vi "e.gate HighSpeedPort Get File - Read Directory.vi"(7 "Timeout (ms) [1000]":i32=1000, 8 "error in (no error)":errorcluster, 10 "Drive Index":T1(ring), 11 "Configuration in":T2) -> (0 "error out":errorcluster, 2 "data out":string[](array[string]), 3 "Configuration out":T2)   [LabVIEW 2016]
uses:
  e.gate Configuration.ctl
  e.gate Channel Data.ctl
  e.gate Data Type.ctl
  e.gate Protocol Type.ctl
  e.gate Module  Data.ctl
  e.gateHSP_DLLhandle.ctl
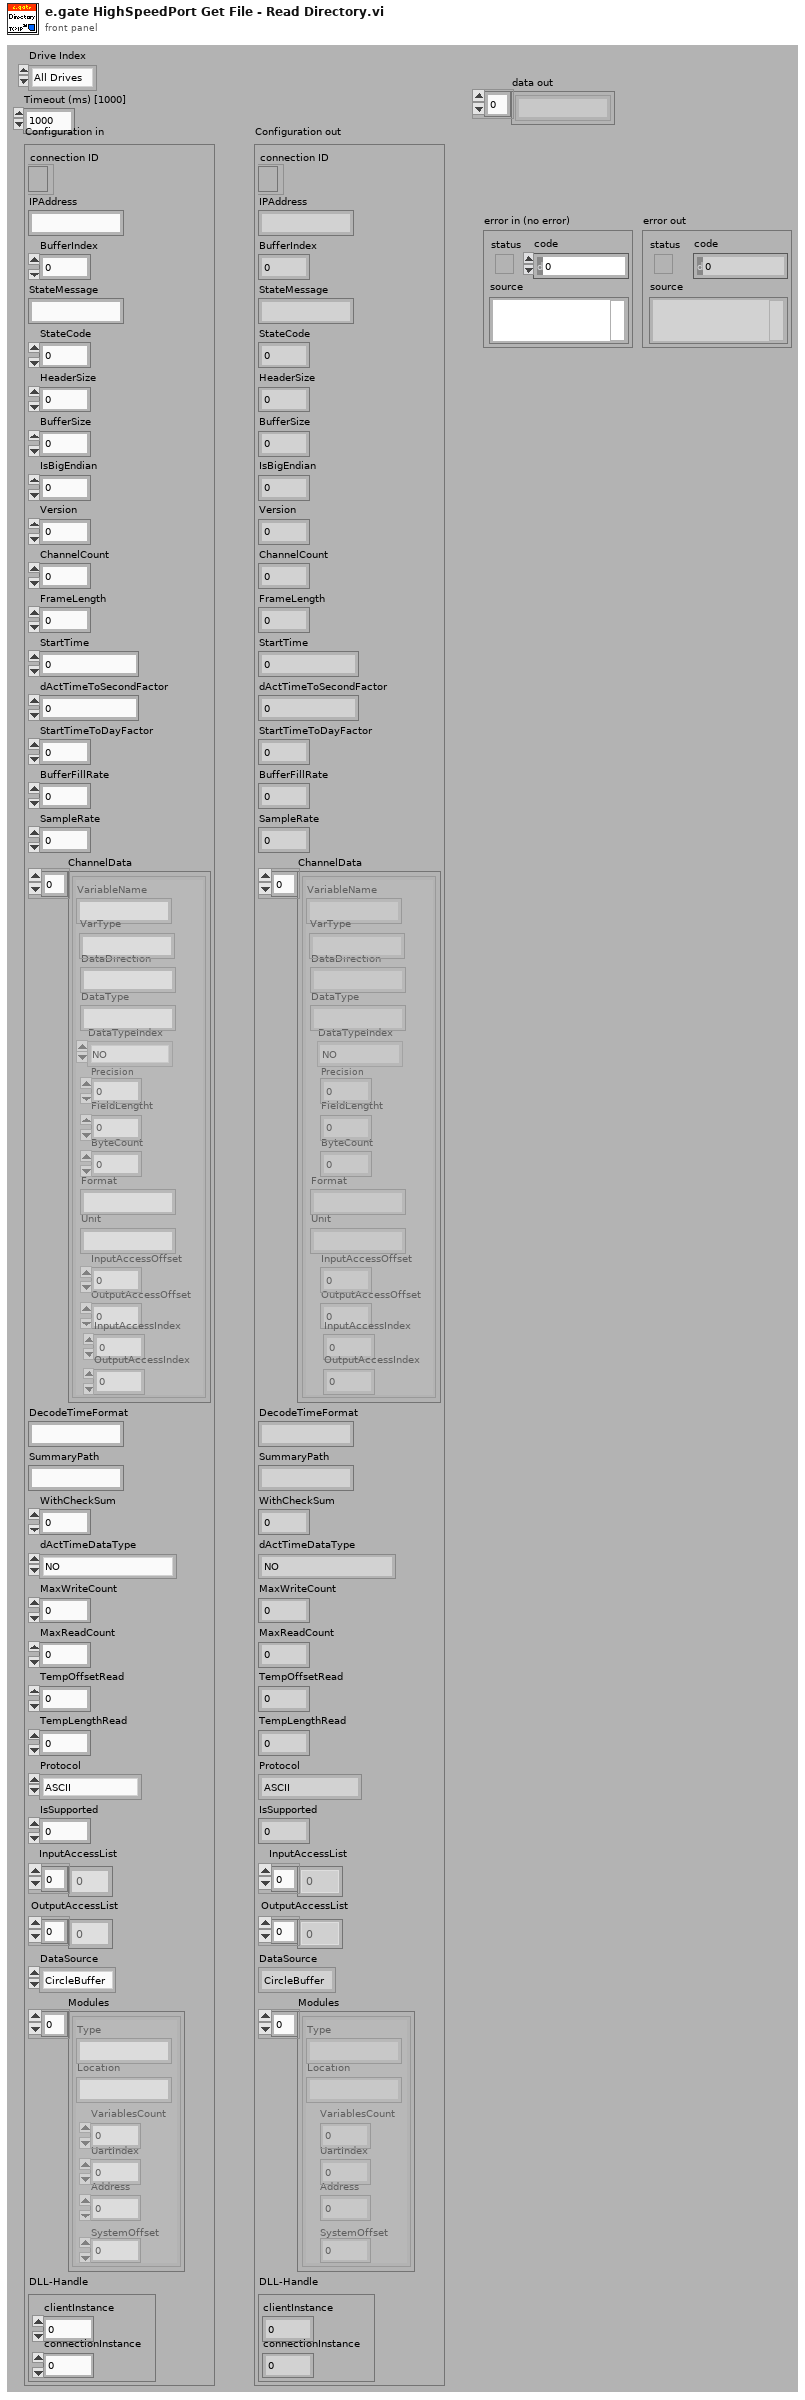
[diagram p1: front panel]
types:
  T1 = enum16{"All Drives", "Flash - Application Files", "Flash - Data", "USB Storage - Data", "Virtual State", "Virtual Circlebuffer", "Virtual Onlinebuffer", "Virtual Archive", "Virtual Logger"}
  T2 = typedef "e.gate Configuration.ctl" = cluster{"connection ID":refnum<k5>, "IPAddress":string, "BufferIndex":i32, "StateMessage":string, "StateCode":i8, "HeaderSize":i32, "BufferSize":i32, "IsBigEndian":i32, "Version":i32, "ChannelCount":i32, "FrameLength":i32, "StartTime":dbl, "dActTimeToSecondFactor":dbl, "StartTimeToDayFactor":dbl, "BufferFillRate":dbl, "SampleRate":dbl, "ChannelData":T3[], "DecodeTimeFormat":string, "SummaryPath":string, "WithCheckSum":i32, "dActTimeDataType":T4, "MaxWriteCount":i32, "MaxReadCount":i32, "TempOffsetRead":i32, "TempLengthRead":i32, "Protocol":T5, "IsSupported":i32, "InputAccessList":i32[], "OutputAccessList":i32[], "DataSource":enum16{"CircleBuffer", "test.con Logger", "test.con Archive"}, "Modules":T6[], "DLL-Handle":T7}
  T3 = typedef "e.gate Channel Data.ctl" = cluster{"VariableName":string, "DataDirection":string, "DataType":string, "DataTypeIndex":T4, "Precision":i16, "FieldLengtht":i16, "ByteCount":i32, "Format":string, "Unit":string, "InputAccessOffset":i32, "OutputAccessOffset":i16, "InputAccessIndex":i16, "OutputAccessIndex":i16, "VarType":string}
  T4 = typedef "e.gate Data Type.ctl" = enum16{"NO", "BOOL", "SINT8", "USINT8", "SINT16", "USINT16", "SINT32", "USINT32", "FLOAT", "SET8", "SET16", "SET32", "DOUBLE", "SINT64", "USINT64", "SET64"}
  T5 = typedef "e.gate Protocol Type.ctl" = enum16{"ASCII", "HighspeedPort Online", "HighspeedPort Buffer", "eGateHighspeedPortDLL "}
  T6 = typedef "e.gate Module  Data.ctl" = cluster{"Type":string, "Location":string, "VariablesCount":i16, "UartIndex":i16, "Address":i16, "SystemOffset":i16}
  T7 = typedef "e.gateHSP_DLLhandle.ctl" = cluster{"clientInstance":i32, "connectionInstance":i32}
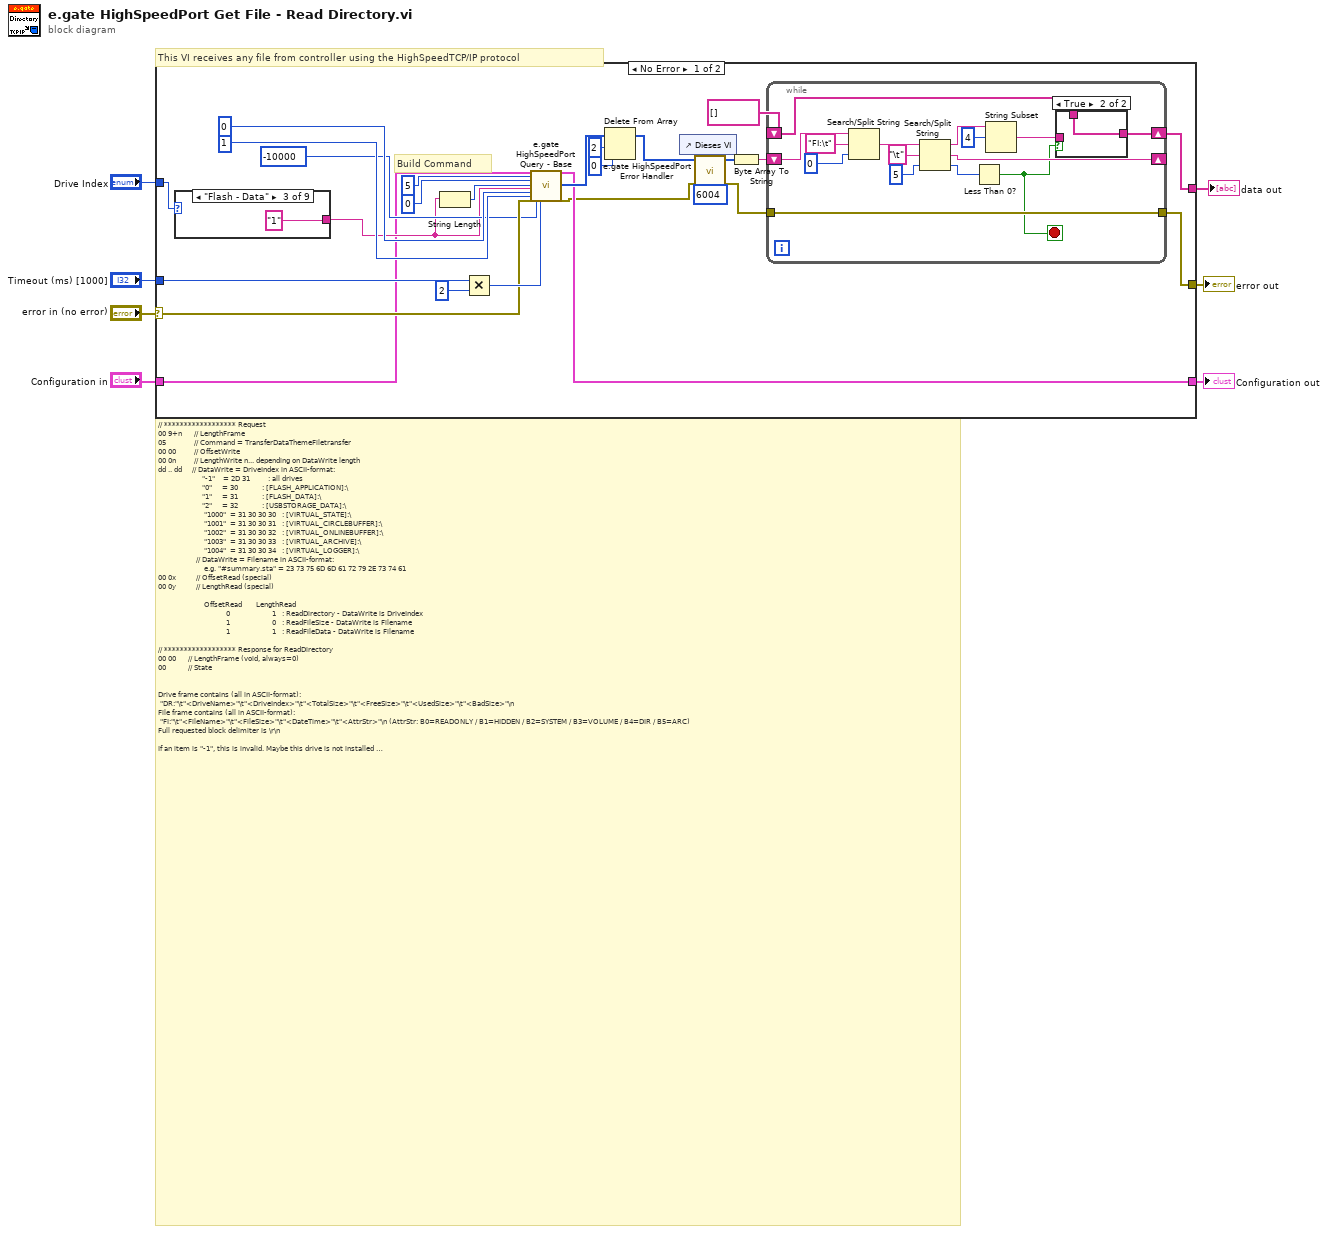
[diagram p0: block diagram]
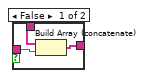
[diagram p2: hidden frame]
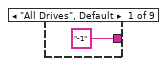
[diagram p3: hidden frame]
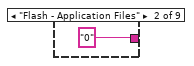
[diagram p4: hidden frame]
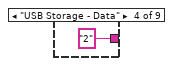
[diagram p5: hidden frame]
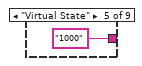
[diagram p6: hidden frame]
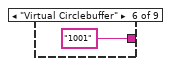
[diagram p7: hidden frame]
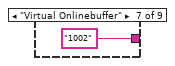
[diagram p8: hidden frame]
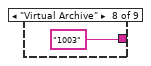
[diagram p9: hidden frame]
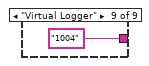
[diagram p10: hidden frame]
diagram:
  # "// ****************** Request\n00 9+n\t\t\t\t\t\t// LengthFrame\n05\t\t\t\t\t\t\t       // Command = TransferDataThemeFiletransfer\n00 00\t\t\t\t   \t\t// OffsetWrite\n00 0n\t\t\t\t\t   \t// LengthWrite n... depending on DataWrite length\ndd .. dd\t\t\t\t\t// DataWrite = DriveIndex in ASCII-format:\n\t\t\t\t\t\t\t              \t\"-1\"    = 2D 31         : all drives\n\t\t\t\t\t\t              \t\t\"0\"     = 30            : [FLASH_APPLICATION]:\\\n\t\t\t\t\t\t\t              \t\"1\"     = 31            : [FLASH_DATA]:\\\n\t\t\t              \t\t\t\t\t\"2\"     = 32            : [USBSTORAGE_DATA]:\\\n\t\t\t\t\t\t               \t\t\"1000\"  = 31 30 30 30   : [VIRTUAL_STATE]:\\\n\t\t\t\t\t\t\t               \t\"1001\"  = 31 30 30 31   : [VIRTUAL_CIRCLEBUFFER]:\\\n\t\t\t\t\t\t\t               \t\"1002\"  = 31 30 30 32   : [VIRTUAL_ONLINEBUFFER]:\\\n\t\t\t\t\t\t               \t\t\"1003\"  = 31 30 30 33   : [VIRTUAL_ARCHIVE]:\\\n\t\t\t\t\t\t               \t\t\"1004\"  = 31 30 30 34   : [VIRTUAL_LOGGER]:\\\n\t\t\t\t\t\t            \t// DataWrite = Filename in ASCII-format:\n\t\t\t\t\t\t\t               \te.g. \"#summary.sta\" = 23 73 75 6D 6D 61 72 79 2E 73 74 61\n00 0x\t\t\t\t\t\t    // OffsetRead (special)\n00 0y\t\t\t\t\t\t    // LengthRead (special)\n\n\t\t\t\t\t\t\t\t               OffsetRead      \tLengthRead\n\t\t\t\t\t\t\t                          \t0\t                  \t\t1\t\t\t: ReadDirectory - DataWrite is DriveIndex\n\t\t\t\t\t\t\t                          \t1\t\t                  \t0\t\t\t: ReadFileSize - DataWrite is Filename\n\t\t\t\t\t\t\t                          \t1\t\t\t                  1\t\t\t: ReadFileData - DataWrite is Filename\n\n// ****************** Response for ReadDirectory\n00 00\t\t\t\t\t\t// LengthFrame (void, always=0)\n00\t\t\t\t\t    \t\t// State\n\n\nDrive frame contains (all in ASCII-format):\n\t\"DR:\"\\t\"<DriveName>\"\\t\"<DriveIndex>\"\\t\"<TotalSize>\"\\t\"<FreeSize>\"\\t\"<UsedSize>\"\\t\"<BadSize>\"\\n\nFile frame contains (all in ASCII-format):\n\t\"FI:\"\\t\"<FileName>\"\\t\"<FileSize>\"\\t\"<DateTime>\"\\t\"<AttrStr>\"\\n\t(AttrStr: B0=READONLY / B1=HIDDEN / B2=SYSTEM / B3=VOLUME / B4=DIR / B5=ARC)\nFull requested block delimiter is \\r\\n\n\nIf an item is \"-1\", this is invalid. Maybe this drive is not installed or parameter is not available there !!!\n\ne.g. ReadDirectory of DriveIndex=0:\n\\x00\\x00\\x00\nDR:\\t[FLASH_APPLICATION]:\\\\t0\\t7077888\\t4878336\\t2199552\\t0\\n\nFI:\\tecpu01.bin\\t1764336\\t2008-03-11\\t10:51:40\\t0020\\n\nFI:\\tecpu01.ini\\t495\\t1980-01-01\\t12:00:00\\t0020\\n\nFI:\\tconfig.sys\\t219\\t1980-01-01\\t12:00:00\\t0020\\n\nFI:\\tfpga.bit\\t403014\\t1980-01-01\\t12:00:00\\t0020\\n\nFI:\\tftp_lic.cnf\\t538\\t2008-02-26\\t15:43:42\\t0020\\n\nFI:\\tmaster.gcf\t10750\\t2008-02-26\\t15:43:50\\t0020\\n\nFI:\\tself.ini\\t78\\t2008-03-11 09:27:36\\t0020\\n\\r\\n\n\n// ****************** Response for ReadFileSize\n00 1+n\t\t\t\t\t\t// LengthFrame\n00\t\t\t\t\t\t       \t// State\ndd .. dd\t\t\t\t\t// DataRead: Size of file in ASCII-format with length n\n\n// ****************** Response for ReadFileData\n00 1+n\t\t\t\t\t\t// LengthFrame\n00\t\t\t\t\t\t       \t// State\ndd .. dd\t\t\t\t\t// DataRead: Content of file with length n\n\n\nATTENTION: If LengthFrame is 0xFFFF, an ExtendedLengthFrame element with 4 bytes is inserted after LF LF, to make possible,\n\tto transfer more than 65534 bytes of data !!!"
  # "This VI receives any file from controller using the HighSpeedTCP/IP protocol"
  n1 = case shown="No Error" "error in (no error)" {
    selector: "error in (no error)" -> [w28 w63]
    tunnel: [w18 w64] -> w6
    tunnel: "Configuration in" -> [w19 w64]
    tunnel: [w11 w63] -> w3
    tunnel: "Timeout (ms) [1000]" -> [w34 _]
    tunnel: "Drive Index" -> [w25 _]
    tunnel: [w9 _] -> w1
    frame No Error {
      # "Build Command"
      n2 = case shown="\"Flash - Data\"" w25 {
        tunnel: ["-1" "0" "1" "2" "1000" "1001" "1002" "1003" "1004"] -> w22
        frame "All Drives", Default {
        }
        frame "Flash - Application Files" {
        }
        frame "Flash - Data" {
        }
        frame "USB Storage - Data" {
        }
        frame "Virtual State" {
        }
        frame "Virtual Circlebuffer" {
        }
        frame "Virtual Onlinebuffer" {
        }
        frame "Virtual Archive" {
        }
        frame "Virtual Logger" {
        }
      }
      n3 = String Length(string=w22) -> (length=w29:i32)
      n4 = Multiply(x=w34, y=2) -> (x*y=w32:i32)
      n5 = call "e.gate HighSpeedPort Query - Base.vi"("e.gate Configuration in"=w19, "Command"=5, "OffsetWrite"=0 ("Command"), "LengthWrite"=w29, "DataWrite"=w22, "OffsetRead"=0 ("Command"), "LengthRead"=1 ("Command"), "error in (no error)"=w28, "TCP LengthReadt"=-10000, "Timeout (1000)"=w32) -> ("e.gate Configuration out"=w18:T2, "Data (out binary)"=w23:u8[], "error out"=w14:errorcluster)  [unwired: 15 out]
      n6 = Delete From Array(array=w23, length=2, index=0) -> (array with subset deleted=w15:u8[])  [unwired: 1 out]
      n7 = control-ref of="Dieses VI"() -> (w16:refnum<vi>)
      n8 = call "e.gate HighSpeedPort Error Handler.vi"("error code start index"=6004, "VI reference"=w16, "error in (no error)"=w14, "binary data in"=w15) -> ("error out"=w10:errorcluster, "binary out"=w13:u8[])  [unwired: 6 out]
      n9 = Byte Array To String(unsigned byte array=w13) -> (string=w12:string)
      n10 = while {
        tunnel: w10 -> [w43]
        tunnel: [w43] -> w11
        shift-right: [w42] -> _
        shift-left: w12 -> [w49]
        shift-right: [w41] -> w9
        shift-left: string[] [] -> [w40]
        stop <- w35 stop-if-true
        n11 = Search/Split String(string=w49, search string/char (-)="FI:\t" ("Nach String/Zeichen suchen (-)"), offset (0)=0 ("Offset (0)")) -> (match + rest of string=w46:string)  [unwired: 2 out]
        n12 = Search/Split String(string=w46, search string/char (-)="\t" ("Nach String/Zeichen suchen (-)"), offset (0)=5 ("Offset (0)")) -> (substring before match=w38:string, match + rest of string=w42:string, offset of match=w39:i32)
        n13 = Less Than 0?(x=w39) -> (x < 0?=w35:bool)
        n14 = String Subset(string=w38, offset (0)=4 ("Offset (0)")) -> (substring=w37:string)  [unwired: 1 out]
        n15 = case shown="True" w35 {
          tunnel: [w52 w53] -> w41
          tunnel: w40 -> [w51 w53]
          tunnel: w37 -> [w50 _]
          frame False {
            n16 = Build Array (concatenate)(w51, w50) -> (w52:string[])
          }
          frame True {
          }
        }
      }
    }
    frame Error {
    }
  }
  "Configuration out" <- w6
  "error out" <- w3
  "data out" <- w1
